vi "SCAN FROM STRING.vi"() -> ()   [LabVIEW 2019]
panel:
  out "output 3":i32
  out "output 2":string
  out "output 1":string
  in  "String":string="MY NAME IS SURAKSHITH AND I LIVE IN COIMBATORE .MY AGE IS 20."
  # "SCAN FROM STRING"
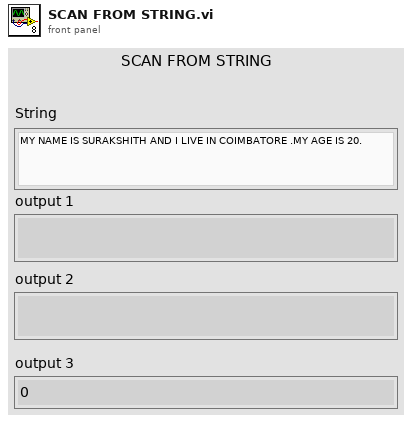
[diagram p1: front panel]
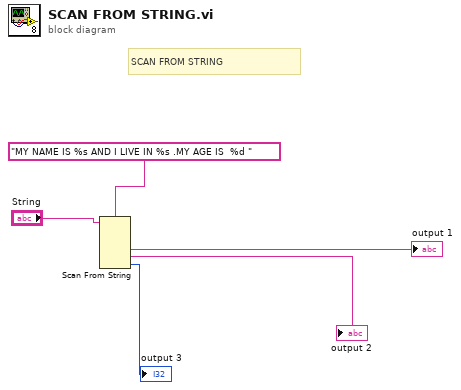
[diagram p0: block diagram]
diagram:
  # "SCAN FROM STRING"
  n1 = Scan From String(format string="MY NAME IS %s AND I LIVE IN %s .MY AGE IS  %d " ("String"), input string="String") -> (output 1=→"output 1":string, output 2=→"output 2":string, output 3=→"output 3":i32)  [unwired: 5 in, 3 out]
